vi "HFRR ADV v04 new software.vi"() -> ()   [LabVIEW 2025] (continued)
                        n2285 = property on="Coefficient of Friction" class="WFChart (strict)"("History Data"=w3332) -> ()  [unwired: 2 in, 2 out]
                        n2286 = property on="Frictional Force ( N )" class="WFChart (strict)"("History Data"=w3332) -> ()  [unwired: 2 in, 2 out]
                        n2287 = property on="Electrical Contact Resistance ( % )" class="WFChart (strict)"("History Data"=w3332) -> ()  [unwired: 2 in, 2 out]
                        n2288 = property on="Humidity ( %RH )" class="WFChart (strict)"("History Data"=w3332) -> ()  [unwired: 2 in, 2 out]
                        n2289 = property on="Stroke ( mm )" class="WFChart (strict)"("History Data"=w3333) -> ()  [unwired: 2 in, 2 out]
                        n2290 = property on="Temperature ( Deg C )" class="WFChart (strict)"("History Data"=w3332) -> ()  [unwired: 2 in, 2 out]
                        n2291 = property on="Service Password Log" class="Str"("Visible"=w3334) -> ()  [unwired: 2 in, 2 out]
                        n2292 = property on="Password 3" class="Clust (strict)"("Visible"=w3334) -> ()  [unwired: 2 in, 2 out]
                      }
                    }
                    "TEST FILE NAM,E SAVED" <- TRUE ("TEST FILE NAM,E SAVED")
                  }
                }
              }
            }
          }
        }
        n2293 = case shown="True" w2651 {
          frame False {
            n2294 = local write "tfalg"(0.0 ("tfalg")) -> ()
          }
          frame True {
            n2295 = local read "tfalg"() -> (w2796:dbl)
            n2296 = Equal?(x=w2796, y=0.0) -> (x = y?=w2797:bool)
            n2297 = case shown="True" w2797 {
              frame False {
              }
              frame True {
                n2298 = local read "Total No. of Tests"() -> (w2800:dbl)
                n2299 = local write "tfalg"(1.0 ("tfalg")) -> ()
                n2300 = local write "acq 2"(FALSE ("acq 2")) -> ()
                n2301 = Wait (ms)(milliseconds to wait=u32 200) -> ()  [unwired: 1 out]
                n2302 = Increment(x=w2800) -> (x+1=w2799:dbl)
                n2303 = local write "Total No. of Tests"(w2799) -> ()
              }
            }
          }
        }
        n2304 = local write "Test \nStatus"(w2657) -> ()
        n2305 = local write "Save"(w2657) -> ()
        n2306 = local read "Main Tab"() -> (w2614:T2)
        n2307 = case shown="True" w2638 {
          tunnel: [FALSE ("RUN") TRUE ("RUN")] -> w2637
          tunnel: [_ 1] -> w2630
          frame False {
          }
          frame True {
          }
        }
        n2308 = In Range and Coerce(upper limit=w2645, x=w2618, lower limit=w2644) -> (In Range?=w2636:bool)  [unwired: 1 out]
        n2309 = In Range and Coerce(upper limit=w2642, x=w2617, lower limit=w2643) -> (In Range?=w2634:bool)  [unwired: 1 out]
        n2310 = case shown="True" w2650 {
          frame False {
            n2311 = local read "Rt 3"() -> (w2778:bool)
            n2312 = case shown="True" w2778 {
              frame False {
              }
              frame True {
                n2313 = local write "Rt 3"(FALSE ("Rt 3")) -> ()
                n2314 = local write "Json End Flg"(TRUE ("Upld AR 2")) -> ()
              }
            }
            "Rt" <- TRUE ("Rt")
            "Rt 2" <- FALSE ("Rt")
          }
          frame True {
            n2315 = local read "Rt"() -> (w2785:bool)
            n2316 = local write "Rt 2"(TRUE ("Rt 2")) -> ()
            n2317 = case shown="True" w2785 {
              frame False {
              }
              frame True {
                w2786 = TRUE ("Upld AR 2")
                n2318 = local write "Rt"(FALSE ("Rt")) -> ()
                n2319 = local write "Upld AR"(w2786) -> ()
                n2320 = local write "Json St Flg"(w2786) -> ()
              }
            }
            "Rt 3" <- TRUE ("Rt 3")
          }
        }
        n2321 = case shown="True" w2636 {
          tunnel: [FALSE ("RUN") TRUE ("RUN")] -> w2635
          tunnel: [_ 2] -> w2629
          frame False {
          }
          frame True {
          }
        }
        n2322 = case shown="True" w2634 {
          tunnel: [FALSE ("RUN") TRUE ("RUN")] -> w2633
          tunnel: [_ 3] -> w2628
          frame False {
          }
          frame True {
          }
        }
        n2323 = case shown="\"Acquire\"" w2614 {
          tunnel: w2616 -> [_ w2847]
          frame Default {
            w2846 = 0.0 ("output")
            n2324 = local write "PID-out"(w2846) -> ()
            n2325 = local write "Frequency ( Hz )"(w2846) -> ()
          }
          frame "Acquire" {
            n2326 = stacked-sequence {
              frame #0 {
                n2327 = local read "Auto Start Test"() -> (w2849:bool)
                n2328 = case shown="True" w2849 {
                  tunnel: "RUN" -> [w2870 w2873]
                  tunnel: [w2870 w2872] -> w2850
                  frame False {
                  }
                  frame True {
                    n2329 = local read "Auto Start Temp"() -> (w2871:bool)
                    n2330 = Or(x=w2873, y=w2871) -> (x .or. y?=w2872:bool)
                  }
                }
                n2331 = local read "clk"() -> (w2869:dbl)
                n2332 = local read "Save"() -> (w2865:bool)
                n2333 = Equal?(x=w2869, y=0.0) -> (x = y?=w2866:bool)
                n2334 = And(x=w2866, y=w2865) -> (x .and. y?=w2867:bool)
                n2335 = Not(x="Engage") -> (.not. x?=w2856:bool)
                n2336 = case shown="True" w2850 {
                  tunnel: [0.0 w2890] -> w2852
                  frame False {
                    (unwired) TRUE ("Visible")
                    n2337 = local read "Auto Start Test"() -> (w2877:bool)
                    n2338 = local write "Start Time"(TRUE ("Start Time")) -> ()
                    n2339 = property on="Stroke 2" class="DigNum (strict)"("Visible"=FALSE) -> ()  [unwired: 2 in, 2 out]
                    n2340 = case shown="False" w2877 {
                      frame False {
                        n2341 = property on="Heater Button" class="Bool (strict)"("DisabledEnum"=T13."Enabled" ("Disabled")) -> ()  [unwired: 2 in, 2 out]
                        n2342 = property on="Humidity" class="Bool (strict)"("DisabledEnum"=T13."Enabled" ("Disabled")) -> ()  [unwired: 2 in, 2 out]
                      }
                      frame True {
                      }
                    }
                    n2343 = case shown="False" "TestCompFlg" {
                      frame False {
                        n2344 = local read "StartFlg"() -> (w2885:bool)
                        n2345 = case shown="True" w2885 {
                          frame False {
                          }
                          frame True {
                            n2346 = flat-sequence {
                              frame #0 {
                                n2347 = local read "EVENT LOG"() -> (w2887:string)
                                n2348 = call "Event Log.vi"("Content"="Test was interrupted", "EVENT LOG"=w2887) -> ("EVENT LOG"=w2888:string)  [unwired: 8 in, 1 out]
                                n2349 = local write "EVENT LOG"(w2888) -> ()
                              }
                              frame #1 {
                                w2889 = FALSE ("StartFlg")
                                n2350 = local write "Heater Button"(w2889) -> ()
                                n2351 = local write "StartFlg"(w2889) -> ()
                                n2352 = local write "Humidity"(w2889) -> ()
                              }
                            }
                          }
                        }
                      }
                      frame True {
                      }
                    }
                    n2353 = local write "String 14"("Test will autostart once parameters reach the set value." ("String 14")) -> ()
                  }
                  frame True {
                    (unwired) FALSE ("Visible")
                    n2354 = property on="Stroke 2" class="DigNum (strict)"("Visible"=TRUE) -> ()  [unwired: 2 in, 2 out]
                    n2355 = property on="STOP 2" class="Bool (strict)"("Disabled"=u8 2) -> ()  [unwired: 2 in, 2 out]
                    n2356 = local write "String 14"(" Running....." ("String 14")) -> ()
                    n2357 = property on="Heater Button" class="Bool (strict)"("DisabledEnum"=T13."Disabled and Grayed Out" ("Disabled")) -> ()  [unwired: 2 in, 2 out]
                    n2358 = property on="Humidity" class="Bool (strict)"("DisabledEnum"=T13."Disabled and Grayed Out" ("Disabled")) -> ()  [unwired: 2 in, 2 out]
                    n2359 = case shown="True" "Start Time" {
                      selector: "Start Time" -> [_ w2903]
                      frame False {
                      }
                      frame True {
                        n2360 = Not(x=w2903) -> (.not. x?=w2902:bool)
                        n2361 = local write "Start Time"(w2902) -> ()
                        n2362 = local read "EVENT LOG"() -> (w2904:string)
                        n2363 = call "Event Log.vi"("Content"="Test in progress", "EVENT LOG"=w2904) -> ("EVENT LOG"=w2906:string)  [unwired: 8 in, 1 out]
                        n2364 = local write "EVENT LOG"(w2906) -> ()
                      }
                    }
                    n2365 = local read "Set Hz"() -> (w2900:dbl)
                    n2366 = call <vilib>:"Uniform White Noise Waveform.vi"() -> ("signal out"=w2899:waveform(dbl))  [unwired: 10 in, 1 out]
                    n2367 = Add(x=w2900, y=w2899) -> (x+y=w2898:waveform(dbl))
                    n2368 = Multiply(x=w2898, y=ext 0.1) -> (x*y=w2890:waveform(ext))
                    "StartFlg" <- TRUE ("StartFlg")
                  }
                }
                n2369 = case shown="True" w2867 {
                  frame False {
                  }
                  frame True {
                    n2370 = local write "clk"(10.0 ("clk")) -> ()
                    n2371 = Get Date/Time In Seconds() -> (seconds since 1Jan1904=w2909:timestamp)
                    n2372 = To Double Precision Float(number=w2909) -> (double precision float=w2907:dbl)
                    n2373 = local write "acq timer"(w2907) -> ()
                    n2374 = local write "act save time"(w2907) -> ()
                  }
                }
                n2375 = call "Elapsed Time"("Time Target (s)"="Countdown", "Reset"=w2856) -> ("Elapsed Time (s)"=w2861:dbl, "Time has Elapsed"=w2859:bool)  [unwired: 10 in, 6 out]
                "Countdown 2" <- w2861
                n2376 = Subtract(x=w2861, y=2.0) -> (x-y=w2864:dbl)
                n2377 = Less?(x=w2864, y="Countdown") -> (x < y?=w2862:bool)
                n2378 = And(x=w2862, y=w2859) -> (x .and. y?=w2858:bool)
                n2379 = case shown="True" w2858 {
                  frame False {
                  }
                  frame True {
                    (unwired) dbl[] [] ("History Data")
                    n2380 = local write "Engage"(FALSE ("Engage")) -> ()
                    n2381 = local write "RUN"(TRUE ("RUN")) -> ()
                    n2382 = local read "Humidity ( %RH )"() -> (→"Rh Before":dbl)
                  }
                }
                n2383 = local read "Test \nStatus"() -> (w2854:bool)
                n2384 = Select(t=w2852, s=w2854, f=0.0) -> (s? t:f=w2853:dbl)
                n2385 = local write "Frequency ( Hz )"(w2853) -> ()
              }
              frame #1 {
                w2932 = 1000000.0 ("x")
                # "HC;1/0\nST;VALUE"
                # "Elapsed time\ncof\nstroke\nAir temp\nTemp\nHumidity"
                # "acq timer\n\nact save time"
                # "convert to microseconds"
                n2386 = local read "COUNT"() -> (w2915:i32)
                n2387 = local read "Rate"() -> (w2928:dbl)
                n2388 = Divide(x=w2932, y=w2928) -> (x/y=w2933:dbl)
                n2389 = Greater Or Equal?(x=w2915, y=250) -> (x >= y?=w2914:bool)
                n2390 = Get Date/Time In Seconds() -> (seconds since 1Jan1904=w2935:timestamp)
                n2391 = case shown="True" w2914 {
                  frame False {
                    n2392 = local read "COUNT"() -> (w2936:i32)
                    n2393 = Increment(x=w2936) -> (x+1=w2937:i32)
                    n2394 = local write "COUNT"(w2937) -> ()
                  }
                  frame True {
                    n2395 = local write "COUNT"(0 ("COUNT")) -> ()
                  }
                }
                n2396 = local read "Samplingtime 2"() -> (w2913:dbl)
                n2397 = local read "act save time"() -> (w2930:dbl)
                n2398 = Divide(x=w2933, y=w2932) -> (x/y=w2931:dbl)
                n2399 = To Double Precision Float(number=w2935) -> (double precision float=w2924:dbl)
                n2400 = Add(x=w2930, y=w2913) -> (x+y=w2929:dbl)
                n2401 = local read "acq timer"() -> (w2934:dbl)
                n2402 = local read "COUNT"() -> (w2917:i32)
                n2403 = Greater Or Equal?(x=w2924, y=w2929) -> (x >= y?=w2912:bool)
                n2404 = Multiply(x=w2931, y=w2917) -> (x*y=w2923:dbl)
                n2405 = Subtract(x=w2924, y=w2934) -> (x-y=w2926:dbl)
                n2406 = local read "Save"() -> (w2927:bool)
                n2407 = Add(x=w2926, y=w2923) -> (x+y=w2910:dbl)
                "Elapsed time 3" <- w2910
                n2408 = And(x=w2912, y=w2927) -> (x .and. y?=w2925:bool)
                n2409 = Divide(x=w2910, y=60.0) -> (x/y=w2921:dbl)
                n2410 = local read "Test \nStatus"() -> (w2911:bool)
                n2411 = local read "clk"() -> (w2918:dbl)
                n2412 = Equal?(x=w2918, y=10.0) -> (x = y?=w2920:bool)
                n2413 = case shown="True" w2925 {
                  tunnel: w2924 -> [_ w3040]
                  tunnel: [FALSE ("Boolean 2") TRUE ("Boolean 2")] -> _
                  frame False {
                  }
                  frame True {
                    w2994 = ";" ("Substring")
                    # "Pid out/\nFreq response value"
                    n2414 = local write "act save time"(w3040) -> ()
                    n2415 = local read "FILE"() -> (w2988:string)
                    n2416 = call "file check.vi"("file name in"=w2988) -> ("error out"=w2991:errorcluster, "file name out"=w2986:string)  [unwired: 9 in]
                    n2417 = call "FILE PATH CREATION.vi"("error in"=w2991, "FILE NAME :"=w2986) -> ("FILE OUT"=w2989:path)  [unwired: 8 in, 1 out]
                    n2418 = Concatenate Strings(w2986, ".dgf" ("Substring")) -> (w2990:string)
                    n2419 = local read "FF 2"() -> (→"Frictional Force ( N )" →"Frictional Force ( N )":dbl)
                    n2420 = Build Path(base path=w2989, name or relative path=w2990) -> (appended path=w2985:path)
                    n2421 = local read "COF 2"() -> (w2999:dbl)
                    "cof" <- w2999
                    "Coefficient of Friction" <- w2999
                    "COF 4" <- w2999
                    "Coefficient of Friction" <- w2999
                    n2422 = local read "TEMP"() -> (w3002:dbl)
                    "Temp" <- w3002
                    "Temperature ( Deg C )" <- w3002
                    n2423 = local read "Humidity ( %RH )"() -> (w3001:dbl)
                    "Humidity ( %RH )" <- w3001
                    "Humidity ( %RH )" <- w3001
                    n2424 = local read "Frequency ( Hz )"() -> (w3008:dbl)
                    n2425 = local read "Elapsed time"() -> (w3033:dbl)
                    n2426 = local read "AIR TEMP"() -> (w3006:dbl)
                    n2427 = local read "PID-out"() -> (w3011:dbl)
                    n2428 = local write "Temperature ( Deg C )"(w3002) -> ()
                    n2429 = Number To Fractional String(number="measured_stroke", width (-)=i16 9 ("precision (6)"), precision (6)=i16 6) -> (F-format string=w3026:string)  [unwired: 1 in]
                    n2430 = Number To Fractional String(number=w3006, width (-)=i16 9 ("precision (6)"), precision (6)=i16 3) -> (F-format string=w3025:string)  [unwired: 1 in]
                    n2431 = Number To Fractional String(number=w3002, width (-)=i16 9 ("precision (6)"), precision (6)=i16 3) -> (F-format string=w3022:string)  [unwired: 1 in]
                    n2432 = Number To Fractional String(number=w3001, width (-)=i16 9 ("precision (6)"), precision (6)=i16 3) -> (F-format string=w3019:string)  [unwired: 1 in]
                    n2433 = Number To Fractional String(number=0.0, width (-)=i16 9 ("precision (6)"), precision (6)=i16 3) -> (F-format string=w3016:string)  [unwired: 1 in]
                    n2434 = Number To Fractional String(number=w3011, width (-)=i16 9 ("precision (6)"), precision (6)=i16 3) -> (F-format string=w3012:string)  [unwired: 1 in]
                    n2435 = Number To Fractional String(number=w3008, width (-)=i16 9 ("precision (6)"), precision (6)=i16 3) -> (F-format string=w3007:string)  [unwired: 1 in]
                    n2436 = Number To Fractional String(number=w2999, width (-)=i16 9 ("precision (6)"), precision (6)=i16 6) -> (F-format string=w3034:string)  [unwired: 1 in]
                    n2437 = Number To Fractional String(number=w3033, width (-)=i16 14 ("precision (6)"), precision (6)=i16 3) -> (F-format string=w3035:string)  [unwired: 1 in]
                    n2438 = Bundle("y"=1.02, "measured_stroke"="measured_stroke", "y"=0.98) -> (w3000:cluster{"y":dbl, "measured_stroke":dbl, "y":dbl})  [unwired: 1 in]
                    n2439 = Number To Fractional String(number="Ambient Humidity :", width (-)=i16 9 ("precision (6)"), precision (6)=i16 6) -> (F-format string=w2992:string)  [unwired: 1 in]
                    n2440 = local read "RUN"() -> (w2998:bool)
                    n2441 = case shown="True" w2998 {
                      tunnel: w3000 -> [_ w3045]
                      tunnel: "measured_stroke" -> [_ w3044]
                      tunnel: "measured_stroke" -> [_ w3043]
                      tunnel: "measured_stroke" -> [_ w3042]
                      frame False {
                      }
                      frame True {
                        "Stroke ( mm )" <- w3045
                        "Stroke ( mm )" <- w3045
                        "Stroke 4" <- w3044
                        "Stroke 3" <- w3043
                        "Stroke 2" <- w3042
                      }
                    }
                    n2442 = Concatenate Strings(w3035, w2994, w3034, w2994, w3026, w2994, w3025, w2994, w3022, w2994, w3019, w2994, w3016, w2994, w3012, w2994, w3007, w2994, w2992, "\r") -> (w3032:string)
                    n2443 = call <vilib>:"Write Characters To File.vi"("append to file? (new file:F)"=TRUE, "character string"=w3032, "file path (dialog if empty)"=w2985) -> ()  [unwired: 2 in, 1 out]
                    "refresh flag" <- TRUE ("refresh flag")
                  }
                }
                n2444 = case shown="True" w2911 {
                  tunnel: w2921 -> [_ w2947]
                  tunnel: w2926 -> [_ w2957]
                  tunnel: [0.0 w2953] -> _
                  tunnel: w2920 -> [_ w2952]
                  tunnel: [0.0 w2951] -> _
                  tunnel: w2910 -> [_ w2951]
                  tunnel: w2924 -> [w2940 _]
                  frame False {
                    n2445 = local write "acq timer"(w2940) -> ()
                    n2446 = local write "Test Duration Status"(0.0 ("Test Duration Status")) -> ()
                  }
                  frame True {
                    n2447 = local read "Set Hz"() -> (w2954:dbl)
                    n2448 = local write "Elapsed time"(w2947) -> ()
                    n2449 = local read "test time"() -> (w2946:dbl)
                    n2450 = Multiply(x=w2957, y=w2954) -> (x*y=w2956:dbl)
                    n2451 = case shown="False" w2952 {
                      tunnel: w2956 -> [w2958 _]
                      tunnel: [w2958 1.0] -> w2953
                      frame False {
                        n2452 = local write "Cycles elapsed"(w2958) -> ()
                      }
                      frame True {
                      }
                    }
                    n2453 = Greater?(x=w2947, y=w2946) -> (0:w2955:bool)
                    n2454 = Subtract(x=w2946, y=w2947) -> (x-y=w2945:dbl)
                    "time" <- w2945
                    n2455 = Multiply(x=w2945, y=60.0) -> (x*y=w2944:dbl)
                    n2456 = local write "Time Remaining"(w2944) -> ()
                    n2457 = local write "Remaining Time"(w2944) -> ()
                    n2458 = case shown="True" w2955 {
                      frame False {
                      }
                      frame True {
                        n2459 = stacked-sequence {
                          frame #0 {
                            w2961 = T13."Enabled" ("Disabled")
                            w2960 = FALSE ("TEST FILE NAM,E SAVED")
                            w2964 = "" ("FILE")
                            w2965 = TRUE ("Visible")
                            n2460 = local write "Humidity"(FALSE ("Humidity")) -> ()
                            n2461 = local write "RUN"(FALSE ("OK Button 2")) -> ()
                            n2462 = local write "Heater Button"(FALSE ("Heater Button")) -> ()
                            n2463 = local write "Auto Start Test"(FALSE ("Auto Start Test")) -> ()
                            n2464 = local write "TestCompFlg"(TRUE ("StpFlg")) -> ()
                            n2465 = local read "Humidity ( %RH )"() -> (→"Rh After":dbl)
                            n2466 = property on="STOP 2" class="Bool (strict)"("Disabled"=u8 0) -> ()  [unwired: 2 in, 2 out]
                            n2467 = local read "EVENT LOG"() -> (w2970:string)
                            n2468 = call "Event Log.vi"("Content"="Test Completed", "EVENT LOG"=w2970) -> ("EVENT LOG"=w2969:string)  [unwired: 8 in, 1 out]
                            n2469 = property on="RUN" class="Bool (strict)"("Visible"=w2965) -> ()  [unwired: 2 in, 2 out]
                            n2470 = property on="Auto Start Test" class="Bool (strict)"("Visible"=w2965) -> ()  [unwired: 2 in, 2 out]
                            n2471 = local write "Batch Ref Num :"(w2964) -> ()
                            n2472 = local write "FILE"(w2964) -> ()
                            n2473 = local write "EVENT LOG"(w2969) -> ()
                            n2474 = local write "TEST FILE NAM,E SAVED"(w2960) -> ()
                            n2475 = local write "Fuel Discription :"(w2964) -> ()
                            n2476 = local write "START TEMP"(w2960) -> ()
                            n2477 = local write "Remarks :"(w2964) -> ()
                            n2478 = local write "Main Dashboard Buttons"(T1."Imaging" ("Main Dashboard Buttons")) -> ()
                            n2479 = local write "Main Tab"(T2."Adv Scar" ("Main Tab")) -> ()
                            n2480 = property on="FRICVALZ 2" class="Bool (strict)"("DisabledEnum"=w2961) -> ()  [unwired: 2 in, 2 out]
                            n2481 = property on="FRICVALZ 3" class="Bool (strict)"("DisabledEnum"=w2961) -> ()  [unwired: 2 in, 2 out]
                            n2482 = property on="FRICVALZ 4" class="Bool (strict)"("DisabledEnum"=w2961) -> ()  [unwired: 2 in, 2 out]
                          }
                          frame #1 {
                            n2483 = Wait (ms)(milliseconds to wait=u32 1500) -> ()  [unwired: 1 out]
                          }
                          frame #2 {
                            n2484 = local write "Command"("VC;0") -> ()
                          }
                          frame #3 {
                            n2485 = Wait (ms)(milliseconds to wait=u32 1500) -> ()  [unwired: 1 out]
                          }
                          frame #4 {
                            n2486 = local write "Command"("ST;0") -> ()
                          }
                          frame #5 {
                            n2487 = Wait (ms)(milliseconds to wait=u32 1500) -> ()  [unwired: 1 out]
                          }
                          frame #6 {
                            n2488 = local write "Command"("HE;0") -> ()
                          }
                        }
                      }
                    }
                    n2489 = Divide(x=w2947, y=w2946) -> (x/y=w2950:dbl)
                    n2490 = Multiply(x=w2950, y=100.0) -> (x*y=w2948:dbl)
                    n2491 = local write "Test Duration Status"(w2948) -> ()
                  }
                }
              }
              frame #2 {
                n2492 = case shown="True" "Heater Button" {
                  tunnel: [0.0 ("output") w3068] -> w3046
                  frame False {
                    w3049 = TRUE ("tmpchk")
                    n2493 = local read "TEMP"() -> (w3050:dbl)
                    n2494 = local write "Temp ini"(w3050) -> ()
                    n2495 = local write "Reset 4"(w3049) -> ()
                    n2496 = local write "tmpchk"(w3049) -> ()
                    n2497 = local write "reinit"(TRUE ("reinit")) -> ()
                    n2498 = local write "manual temp log"(TRUE ("manual temp log")) -> ()
                  }
                  frame True {
                    # "Logic to turn off\nthe heater when \ntemp is not rising.\nTime - 60 sec\nDelta t- 5°c"
                    n2499 = local read "Temp ini"() -> (w3057:dbl)
                    n2500 = local read "Auto Start Test"() -> (w3053:bool)
                    n2501 = Less?(x=w3057, y=53.0) -> (x < y?=w3055:bool)
                    n2502 = case shown="False" w3053 {
                      frame False {
                        n2503 = local read "Set Temp"() -> (w3077:dbl)
                        n2504 = local read "TEMP"() -> (w3076:dbl)
                        n2505 = Subtract(x=w3077, y=w3076) -> (x-y=w3075:dbl)
                        n2506 = Absolute Value(x=w3075) -> (abs(x)=w3074:dbl)
                        n2507 = Less?(x=w3074, y=0.5) -> (x < y?=w3072:bool)
                        n2508 = case shown="True" w3072 {
                          tunnel: "manual temp log" -> [_ w3078]
                          frame False {
                          }
                          frame True {
                            n2509 = case shown="True" w3078 {
                              selector: w3078 -> [_ w3079]
                              frame False {
                              }
                              frame True {
                                # "#Event log"
                                n2510 = Not(x=w3079) -> (.not. x?=w3080:bool)
                                n2511 = local write "manual temp log"(w3080) -> ()
                                n2512 = local read "EVENT LOG"() -> (w3083:string)
                                n2513 = call "Event Log.vi"("Content"="Target Temperature reached", "EVENT LOG"=w3083) -> ("EVENT LOG"=w3082:string)  [unwired: 8 in, 1 out]
                                n2514 = local write "EVENT LOG"(w3082) -> ()
                              }
                            }
                          }
                        }
                      }
                      frame True {
                        n2515 = local write "manual temp log"(TRUE ("manual temp log")) -> ()
                      }
                    }
                    n2516 = And(x="tmpchk", y=w3055) -> (x .and. y?=w3058:bool)
                    n2517 = case shown="True" w3058 {
                      frame False {
                      }
                      frame True {
                        n2518 = call "Elapsed Time8"("Time Target (s)"=300.0, "Reset"="Reset 4") -> ("Time has Elapsed"=w3085:bool)  [unwired: 10 in, 7 out]
                        n2519 = flat-sequence {
                          tunnel: w3085 -> [_]
                          frame #0 {
                            n2520 = local write "Reset 4"(FALSE ("Reset 4")) -> ()
                          }
                        }
                        n2521 = case shown="True" w3085 {
                          frame False {
                          }
                          frame True {
                            n2522 = local read "Temp ini"() -> (w3092:dbl)
                            n2523 = Add(x=w3092, y=5.0) -> (x+y=w3090:dbl)
                            n2524 = local read "TEMP"() -> (w3093:dbl)
                            n2525 = Greater?(x=w3093, y=w3090) -> (0:w3091:bool)
                            n2526 = case shown="False" w3091 {
                              frame False {
                                n2527 = local write "Heater Button"(FALSE ("Heater Button")) -> ()
                              }
                              frame True {
                                n2528 = local write "tmpchk"(FALSE ("tmpchk")) -> ()
                              }
                            }
                          }
                        }
                      }
                    }
                    n2529 = local read "Set Temp"() -> (w3066:dbl)
                    n2530 = local read "TEMP"() -> (w3060:dbl)
                    n2531 = call-poly <vilib>:"PID.vi"("reinitialize? (F)"="reinit", "dt (s)"=-1.0, "process variable"=w3060, "setpoint"=w3066) -> ("output"=w3063:dbl)  [unwired: 6 in, 1 out]
                    n2532 = Subtract(x=w3066, y=w3060) -> (x-y=w3067:dbl)
                    n2533 = Add(x=w3066, y=0.5) -> (x+y=w3064:dbl)
                    n2534 = Greater Or Equal?(x=w3060, y=w3064) -> ()  [unwired: 1 out]
                    n2535 = Select(t=0.0, s=FALSE, f=w3063) -> (s? t:f=w3062:dbl)
                    "PID output" <- w3062
                    n2536 = flat-sequence {
                      tunnel: w3062 -> [w3096]
                      tunnel: [w3096] -> w3068
                      frame #0 {
                        n2537 = local write "reinit"(FALSE ("reinit")) -> ()
                      }
                    }
                    n2538 = Bundle(w3067, "output"=w3062, "TEMP"=w3060) -> ()  [unwired: 1 in, 1 out]
                  }
                }
                "PID-out" <- w3046
              }
              frame #3 {
                n2539 = local read "TEMP"() -> (w3098:dbl)
                n2540 = Greater Or Equal?(x=w3098, y="Set Temp 2") -> (x >= y?=w3103:bool)
                n2541 = case shown="True" w3103 {
                  tunnel: [FALSE TRUE] -> w3101
                  frame False {
                  }
                  frame True {
                  }
                }
                "Status 13" <- w3101
                n2542 = And(x=w3101, y="trip1 8") -> (x .and. y?=w3100:bool)
                n2543 = case shown="True" w3100 {
                  frame False {
                    n2544 = local write "Heater Trip Temp"(TRUE ("Heater Trip Temp")) -> ()
                  }
                  frame True {
                    w3106 = FALSE ("OK Button 2")
                    n2545 = case shown="True" "Heater Trip Temp" {
                      selector: "Heater Trip Temp" -> [_ w3108]
                      frame False {
                      }
                      frame True {
                        n2546 = Not(x=w3108) -> (.not. x?=w3107:bool)
                        n2547 = local read "EVENT LOG"() -> (w3111:string)
                        n2548 = local write "Heater Trip Temp"(w3107) -> ()
                        n2549 = call "Event Log.vi"("Content"="Heater Trip", "EVENT LOG"=w3111) -> ("EVENT LOG"=w3110:string)  [unwired: 8 in, 1 out]
                        n2550 = local write "EVENT LOG"(w3110) -> ()
                      }
                    }
                    n2551 = local write "RUN"(w3106) -> ()
                    n2552 = property on="Auto Start Test" class="Bool (strict)"("Value"=w3106) -> ()  [unwired: 2 in, 2 out]
                    n2553 = local write "Heater Button"(w3106) -> ()
                  }
                }
              }
            }
            n2554 = case shown="False" w2847 {
              frame False {
                n2555 = disable-structure shown="Disabled" {
                  frame Disabled {
                    n2556 = stacked-sequence {
                      frame #0 {
                        n2557 = local write "RUN"(FALSE ("OK Button 2")) -> ()
                      }
                      frame #1 {
                      }
                    }
                  }
                  frame Enabled {
                  }
                }
              }
              frame True {
              }
            }
          }
        }
        n2558 = local read "airtempflg"() -> (w2639:bool)
        n2559 = Or(x=w2639, y=w2637) -> (x .or. y?=w2640:bool)
        n2560 = Insert Into Array(array=string[] ["Air Temperature has reached set value,", "Humidity has reached set value,", "Sample Temperaturehas reached set value,", ""], index=0, new element="") -> (w2625:string[])
        n2561 = Build Array(w2630, w2629, w2628) -> (w2626:i32[])
        n2562 = disable-structure shown="Disabled" {
          disable-tunnel: w2640 -> [w2717 _]
          disable-tunnel: w2635 -> [w2716 _]
          disable-tunnel: w2633 -> [w2715 _]
          frame Disabled {
            n2563 = Compound Arithmetic op=AND(w2717, w2716, w2715) -> ()  [unwired: 1 out]
            n2564 = case shown="True" {
              selector: _ -> [_ _]
              frame False {
              }
              frame True {
                w2718 = FALSE ("autostrtflg")
                n2565 = local write "RUN"(TRUE ("RUN")) -> ()
                n2566 = local write "autostrtflg"(w2718) -> ()
                n2567 = local write "autostart"(w2718) -> ()
                n2568 = local write "String 14"(" Running....." ("String 14")) -> ()
              }
            }
          }
          frame Enabled {
          }
        }
        n2569 = for {
          tunnel: w2626 -> [w2768] mode=indexing
          tunnel: w2625 -> [w2767]
          shift-right: [w2764] -> w2624
          shift-left: "" -> [w2766]
          n2570 = Index Array(array=w2767, index=w2768) -> (element=w2765:string)
          n2571 = Concatenate Strings(w2765, w2766) -> (w2764:string)
        }
        n2572 = local write "autostart 2"(w2624) -> ()
        n2573 = local read "Reset Graph"() -> (w2613:bool)
        n2574 = case shown="True" w2613 {
          selector: w2613 -> [_ w2667]
          frame False {
          }
          frame True {
            w2681 = 0.0 ("X Scale.Range:Maximum")
            n2575 = Not(x=w2667) -> (.not. x?=w2666:bool)
            n2576 = local write "Reset Graph"(w2666) -> ()
            n2577 = property on="Electrical Contact Resistance ( % )" class="WFChart (strict)"("XScale.Maximum"=600.0 ("X Scale.Range:Maximum"), "XScale.Minimum"=0.0 ("X Scale.Range:Minimum"), "YScale.Maximum"=100.0 ("Y Scale.Range:Maximum"), "YScale.Minimum"=0.0 ("Y Scale.Range:Minimum")) -> ()  [unwired: 2 in, 2 out]
            n2578 = property on="Frictional Force ( N )" class="WFChart (strict)"("XScale.Maximum"=600.0 ("X Scale.Range:Maximum"), "XScale.Minimum"=0.0 ("X Scale.Range:Minimum"), "YScale.Maximum"=100.0 ("Y Scale.Range:Maximum"), "YScale.Minimum"=0.0 ("Y Scale.Range:Minimum")) -> ()  [unwired: 2 in, 2 out]
            n2579 = property on="Temperature ( Deg C )" class="WFChart (strict)"("XScale.Maximum"=600.0 ("X Scale.Range:Maximum"), "XScale.Minimum"=0.0 ("X Scale.Range:Minimum"), "YScale.Maximum"=100.0 ("Y Scale.Range:Maximum"), "YScale.Minimum"=0.0 ("Y Scale.Range:Minimum")) -> ()  [unwired: 2 in, 2 out]
            n2580 = property on="Humidity ( %RH )" class="WFChart (strict)"("XScale.Maximum"=600.0 ("X Scale.Range:Maximum"), "XScale.Minimum"=0.0 ("X Scale.Range:Minimum"), "YScale.Maximum"=100.0 ("Y Scale.Range:Maximum"), "YScale.Minimum"=0.0 ("Y Scale.Range:Minimum")) -> ()  [unwired: 2 in, 2 out]
            n2581 = property on="Stroke ( mm )" class="WFChart (strict)"("XScale.Maximum"=600.0 ("X Scale.Range:Maximum"), "XScale.Minimum"=0.0 ("X Scale.Range:Minimum"), "YScale.Maximum"=100.0 ("Y Scale.Range:Maximum"), "YScale.Minimum"=0.0 ("Y Scale.Range:Minimum")) -> ()  [unwired: 2 in, 2 out]
            n2582 = property on="Coefficient of Friction" class="WFChart (strict)"("XScale.Maximum"=600.0 ("X Scale.Range:Maximum"), "XScale.Minimum"=0.0 ("X Scale.Range:Minimum"), "YScale.Maximum"=100.0 ("Y Scale.Range:Maximum"), "YScale.Minimum"=0.0 ("Y Scale.Range:Minimum")) -> ()  [unwired: 2 in, 2 out]
            n2583 = property on="Electrical Contact Resistance ( % )" class="WFChart (strict)"("XScale.Minimum"=0.0 ("X Scale.Range:Minimum"), "XScale.Maximum"=600.0 ("X Scale.Range:Maximum"), "YScale.Minimum"=0.0 ("Y Scale.Range:Minimum"), "YScale.Maximum"=100.0 ("Y Scale.Range:Maximum")) -> ()  [unwired: 2 in, 2 out]
            n2584 = property on="Temperature ( Deg C )" class="WFChart (strict)"("XScale.Minimum"=0.0 ("X Scale.Range:Minimum"), "XScale.Maximum"=600.0 ("X Scale.Range:Maximum"), "YScale.Minimum"=0.0 ("Y Scale.Range:Minimum"), "YScale.Maximum"=100.0 ("Y Scale.Range:Maximum")) -> ()  [unwired: 2 in, 2 out]
            n2585 = property on="Coefficient of Friction" class="WFChart (strict)"("XScale.Minimum"=0.0 ("X Scale.Range:Minimum"), "XScale.Maximum"=600.0 ("X Scale.Range:Maximum"), "YScale.Maximum"=1.0 ("X Scale.Range:Minimum"), "YScale.Minimum"=0.0 ("X Scale.Range:Minimum")) -> ()  [unwired: 2 in, 2 out]
            n2586 = property on="Frictional Force ( N )" class="WFChart (strict)"("XScale.Maximum"=600.0 ("X Scale.Range:Maximum"), "XScale.Minimum"=w2681, "YScale.Maximum"=10.0 ("Y Scale.Range:Maximum"), "YScale.Minimum"=w2681) -> ()  [unwired: 2 in, 2 out]
            n2587 = property on="Stroke ( mm )" class="WFChart (strict)"("XScale.Maximum"=600.0 ("X Scale.Range:Maximum"), "XScale.Minimum"=0.0 ("X Scale.Range:Minimum"), "YScale.Maximum"=100.0 ("Y Scale.Range:Maximum"), "YScale.Minimum"=0.0 ("Y Scale.Range:Minimum")) -> ()  [unwired: 2 in, 2 out]
            n2588 = property on="Humidity ( %RH )" class="WFChart (strict)"("XScale.Maximum"=600.0 ("X Scale.Range:Maximum"), "XScale.Minimum"=0.0 ("X Scale.Range:Minimum"), "YScale.Maximum"=100.0 ("Y Scale.Range:Maximum"), "YScale.Minimum"=0.0 ("Y Scale.Range:Minimum")) -> ()  [unwired: 2 in, 2 out]
          }
        }
      }
      frame "Compare Files" {
        # "Elapsed time\ncof\nstroke\nAir temp\nTemp\nHumidity"
        n2589 = case shown="True" "RSTV1 2" {
          frame False {
          }
          frame True {
            n2590 = property on="Humidity ( %RH )" class="XYGraph (strict)"("Y Scale.Display Format:Precision"=u8 0 ("Y Scale.Format & Precision:Precision")) -> ()  [unwired: 2 in, 2 out]
            n2591 = property on="Humidity ( %RH )" class="XYGraph (strict)"("X Scale.Range:Minimum"=0.0, "X Scale.Range:Maximum"=75.0, "Y Scale.Range:Minimum"=48.0, "Y Scale.Range:Maximum"=58.0) -> ()  [unwired: 2 in, 2 out]
          }
        }
        n2592 = case shown="True" "RST CP 2" {
          frame False {
          }
          frame True {
            n2593 = property on="XY Graph 13" class="XYGraph (strict)"("Y Scale.Display Format:Precision"=u8 0 ("Y Scale.Format & Precision:Precision")) -> ()  [unwired: 2 in, 2 out]
            n2594 = property on="XY Graph 13" class="XYGraph (strict)"("X Scale.Range:Minimum"=0.0, "X Scale.Range:Maximum"=75.0, "Y Scale.Range:Minimum"=0.0, "Y Scale.Range:Maximum"=100.0) -> ()  [unwired: 2 in, 2 out]
          }
        }
        n2595 = case shown="True" "RST CP" {
          frame False {
          }
          frame True {
            n2596 = property on="Sample Temperature ( °C )" class="XYGraph (strict)"("Y Scale.Display Format:Precision"=u8 2 ("Y Scale.Format & Precision:Precision")) -> ()  [unwired: 2 in, 2 out]
            n2597 = property on="Sample Temperature ( °C )" class="XYGraph (strict)"("X Scale.Range:Minimum"=0.0, "X Scale.Range:Maximum"=75.0, "Y Scale.Range:Minimum"=58.0, "Y Scale.Range:Maximum"=62.0) -> ()  [unwired: 2 in, 2 out]
          }
        }
        n2598 = case shown="True" "RSTV1 3" {
          frame False {
          }
          frame True {
            n2599 = property on="Air Temperature  ( °C )" class="XYGraph (strict)"("Y Scale.Display Format:Precision"=u8 2 ("Y Scale.Format & Precision:Precision")) -> ()  [unwired: 2 in, 2 out]
            n2600 = property on="Air Temperature  ( °C )" class="XYGraph (strict)"("X Scale.Range:Minimum"=0.0 ("Y Scale.Range:Minimum"), "X Scale.Range:Maximum"=75.0 ("Y Scale.Range:Maximum"), "Y Scale.Range:Minimum"=20.0 ("X Scale.Range:Minimum"), "Y Scale.Range:Maximum"=26.0 ("X Scale.Range:Maximum")) -> ()  [unwired: 2 in, 2 out]
          }
        }
        n2601 = case shown="True" "RSTV1 4" {
          frame False {
          }
          frame True {
            n2602 = property on="Stroke ( mm )" class="XYGraph (strict)"("Y Scale.Display Format:Precision"=u8 2 ("Y Scale.Format & Precision:Precision")) -> ()  [unwired: 2 in, 2 out]
            n2603 = property on="Stroke ( mm )" class="XYGraph (strict)"("X Scale.Range:Minimum"=0.0 ("Y Scale.Range:Maximum"), "X Scale.Range:Maximum"=75.0 ("X Scale.Range:Minimum"), "Y Scale.Range:Minimum"=0.98, "Y Scale.Range:Maximum"=1.02) -> ()  [unwired: 2 in, 2 out]
          }
        }
        n2604 = case shown="True" "rstv2" {
          frame False {
          }
          frame True {
            n2605 = property on="Coefficient Of Friction" class="XYGraph (strict)"("Y Scale.Display Format:Precision"=u8 3 ("Y Scale.Format & Precision:Precision")) -> ()  [unwired: 2 in, 2 out]
            n2606 = property on="Coefficient Of Friction" class="XYGraph (strict)"("X Scale.Range:Minimum"=0.0 ("Y Scale.Range:Maximum"), "X Scale.Range:Maximum"=75.0, "Y Scale.Range:Minimum"=0.0, "Y Scale.Range:Maximum"=1.0 ("X Scale.Range:Minimum")) -> ()  [unwired: 2 in, 2 out]
          }
        }
        n2607 = case shown="True" "RST CP 3" {
          frame False {
          }
          frame True {
            n2608 = property on="Air Temp ( °C ) vs Humidity ( % RH )" class="XYGraph (strict)"("X Scale.Range:Minimum"=18.0, "X Scale.Range:Maximum"=28.0 ("X Scale.Range:Minimum"), "Y Scale.Range:Minimum"=30.0 ("X Scale.Range:Minimum"), "Y Scale.Range:Maximum"=70.0 ("X Scale.Range:Minimum")) -> ()  [unwired: 2 in, 2 out]
          }
        }
        n2609 = case shown="True" "OPEN 1" {
          frame False {
          }
          frame True {
            (unwired) 0  # existing file
            w3387 = "Choose a datalog file to open"  # prompt
            n2610 = local write "OPEN 1"(FALSE ("OPEN 1")) -> ()
            n2611 = String To Path(string="C:\\LAB-IQ\\Data\\") -> (path=w3372:path)
            n2612 = File Dialog(6:"*.dgf" ("pattern"), 7:w3387, 11:w3372) -> (0:w3370:errorcluster, 3:w3378:path)  [unwired: 4 in, 2 out]
            n2613 = Unbundle(w3370) -> ()  [unwired: 3 out]
            n2614 = Strip Path(path=w3378) -> (name=w3377:string)  [unwired: 1 out]
            n2615 = Path To String(path=w3378) -> (string=w3373:string)
            "string1" <- w3373
            n2616 = Match Pattern(string=w3377, regular expression=".dgf") -> (before substring=→"String Control":string)  [unwired: 1 in, 3 out]
            n2617 = Match Pattern(string=w3373, regular expression=".dgf" ("substring (\"\")")) -> (before substring=w3383:string)  [unwired: 1 in, 3 out]
            n2618 = Concatenate Strings(w3383, ".duf" ("Substring")) -> (w3379:string)
            n2619 = String To Path(string=w3379) -> (path=w3384:path)
            n2620 = call <vilib>:"Read Characters From File.vi"("file path (dialog if empty)"=w3384, "start of read offset (chars.:0)"=60 ("start of read offset (chars.: 0)")) -> ("character string"=→"String Control 2":string)  [unwired: 4 in, 3 out]
          }
        }
        n2621 = case shown="True" "OPEN 2" {
          frame False {
          }
          frame True {
            (unwired) 0  # existing file
            w3405 = "Choose a datalog file to open"  # prompt
            n2622 = local write "OPEN 2"(FALSE ("OPEN 1")) -> ()
            n2623 = String To Path(string="C:\\LAB-IQ\\Data\\") -> (path=w3390:path)
            n2624 = File Dialog(6:"*.dgf" ("pattern"), 7:w3405, 11:w3390) -> (0:w3388:errorcluster, 3:w3396:path)  [unwired: 4 in, 2 out]
            n2625 = Unbundle(w3388) -> ()  [unwired: 3 out]
            n2626 = Strip Path(path=w3396) -> (name=w3394:string)  [unwired: 1 out]
            n2627 = Path To String(path=w3396) -> (string=w3391:string)
            "string1 2" <- w3391
            n2628 = Match Pattern(string=w3394, regular expression=".dgf") -> (before substring=→"String Control 3":string)  [unwired: 1 in, 3 out]
            n2629 = Match Pattern(string=w3391, regular expression=".dgf" ("substring (\"\")")) -> (before substring=w3402:string)  [unwired: 1 in, 3 out]
            n2630 = Concatenate Strings(w3402, ".duf" ("Substring")) -> (w3399:string)
            n2631 = String To Path(string=w3399) -> (path=w3397:path)
            n2632 = call <vilib>:"Read Characters From File.vi"("file path (dialog if empty)"=w3397, "start of read offset (chars.:0)"=60 ("start of read offset (chars.: 0)")) -> ("character string"=→"String Control 4":string)  [unwired: 4 in, 3 out]
          }
        }
        n2633 = case shown="True" "OPEN 3" {
          frame False {
          }
          frame True {
            (unwired) 0  # existing file
            w3423 = "Choose a datalog file to open"  # prompt
            n2634 = local write "OPEN 3"(FALSE ("OPEN 1")) -> ()
            n2635 = String To Path(string="C:\\LAB-IQ\\Data\\") -> (path=w3408:path)
            n2636 = File Dialog(6:"*.dgf" ("pattern"), 7:w3423, 11:w3408) -> (0:w3406:errorcluster, 3:w3414:path)  [unwired: 4 in, 2 out]
            n2637 = Unbundle(w3406) -> ()  [unwired: 3 out]
            n2638 = Strip Path(path=w3414) -> (name=w3412:string)  [unwired: 1 out]
            n2639 = Path To String(path=w3414) -> (string=w3409:string)
            "string1 3" <- w3409
            n2640 = Match Pattern(string=w3412, regular expression=".dgf") -> (before substring=→"String Control 5":string)  [unwired: 1 in, 3 out]
            n2641 = Match Pattern(string=w3409, regular expression=".dgf" ("substring (\"\")")) -> (before substring=w3419:string)  [unwired: 1 in, 3 out]
            n2642 = Concatenate Strings(w3419, ".duf" ("Substring")) -> (w3416:string)
            n2643 = String To Path(string=w3416) -> (path=w3420:path)
            n2644 = call <vilib>:"Read Characters From File.vi"("file path (dialog if empty)"=w3420, "start of read offset (chars.:0)"=60 ("start of read offset (chars.: 0)")) -> ("character string"=→"String Control 6":string)  [unwired: 4 in, 3 out]
          }
        }
        n2645 = case shown="True" "OPEN 4" {
          frame False {
          }
          frame True {
            (unwired) 0  # existing file
            w3441 = "Choose a datalog file to open"  # prompt
            n2646 = local write "OPEN 4"(FALSE ("OPEN 1")) -> ()
            n2647 = String To Path(string="C:\\LAB-IQ\\Data\\") -> (path=w3426:path)
            n2648 = File Dialog(6:"*.dgf" ("pattern"), 7:w3441, 11:w3426) -> (0:w3424:errorcluster, 3:w3432:path)  [unwired: 4 in, 2 out]
            n2649 = Unbundle(w3424) -> ()  [unwired: 3 out]
            n2650 = Strip Path(path=w3432) -> (name=w3430:string)  [unwired: 1 out]
            n2651 = Path To String(path=w3432) -> (string=w3427:string)
            "string1 4" <- w3427
            n2652 = Match Pattern(string=w3430, regular expression=".dgf") -> (before substring=→"String Control 7":string)  [unwired: 1 in, 3 out]
            n2653 = Match Pattern(string=w3427, regular expression=".dgf" ("substring (\"\")")) -> (before substring=w3437:string)  [unwired: 1 in, 3 out]
            n2654 = Concatenate Strings(w3437, ".duf" ("Substring")) -> (w3434:string)
            n2655 = String To Path(string=w3434) -> (path=w3438:path)
            n2656 = call <vilib>:"Read Characters From File.vi"("file path (dialog if empty)"=w3438, "start of read offset (chars.:0)"=60 ("start of read offset (chars.: 0)")) -> ("character string"=→"String Control 8":string)  [unwired: 4 in, 3 out]
          }
        }
      }
      frame "About" {
        # "Elapsed time\ncof\nstroke\nmean pos\nTemp\nHumidity"
        n2657 = disable-structure shown="Disabled" {
          frame Disabled {
            n2658 = case shown="True" "Export" {
              frame False {
              }
              frame True {
                w3463 = "                                      " ("string")
                w3465 = "\r"
                (unwired) i16 6 ("width (-)")
                w3542 = "\r"
                w3474 = "\r"
                n2659 = local write "Export"(FALSE ("Export")) -> ()
                n2660 = local read "String 29"() -> (w3511:string)
                n2661 = local read "String 34"() -> (w3499:string)
                n2662 = local read "String 35"() -> (w3494:string)
                n2663 = local read "String 37"() -> (w3490:string)
                n2664 = local read "String 36"() -> (w3487:string)
                n2665 = local read "String 38"() -> (w3484:string)
                n2666 = local read "String 39"() -> (w3481:string)
                n2667 = Match Pattern(string=w3511, regular expression=".dwm") -> (before substring=w3507:string)  [unwired: 1 in, 3 out]
                "before substring" <- w3507
                n2668 = local read "S 38"() -> (w3502:string)
                n2669 = local read "S 39"() -> (w3495:string)
                n2670 = local read "Temperature before test 2"() -> (w3531:dbl)
                n2671 = local read "Temperature after test 2"() -> (w3536:dbl)
                n2672 = local read "Humidity before test 2"() -> (w3517:dbl)
                n2673 = local read "Humidity after test 2"() -> (w3532:dbl)
                n2674 = local read "MWSD 2"() -> (w3528:dbl)
                n2675 = local read "WS1.4 2"() -> (w3544:dbl)
                n2676 = local read "HCF 2"() -> (w3540:dbl)
                n2677 = local read "AVP 2"() -> (w3529:dbl)
                n2678 = Concatenate Strings("1," ("string"), w3502) -> (w3501:string)
                n2679 = Concatenate Strings("2," ("string"), w3499) -> (w3498:string)
                n2680 = Concatenate Strings("3," ("string"), w3495) -> (w3497:string)
                n2681 = Concatenate Strings("4," ("string"), w3494) -> (w3493:string)
                n2682 = Concatenate Strings("5," ("string"), w3490) -> (w3491:string)
                n2683 = Concatenate Strings("6," ("string"), w3487) -> (w3488:string)
                n2684 = Concatenate Strings("7," ("string"), w3484) -> (w3485:string)
                n2685 = Concatenate Strings("8," ("string"), w3481) -> (w3482:string)
                n2686 = local read "Sample ID"() -> (w3549:string)
                n2687 = case shown="\"xlx\"" "Select File Type" {
                  tunnel: w3507 -> [w3552 w3554 w3556]
                  tunnel: [w3550 w3555 w3557] -> w3506
                  frame "xlx" {
                    n2688 = Concatenate Strings(w3552, ".xls" ("string")) -> (w3550:string)
                  }
                  frame "csv" {
                    n2689 = Concatenate Strings(w3554, ".csv" ("string")) -> (w3555:string)
                  }
                  frame "txt" {
                    n2690 = Concatenate Strings(w3556, ".txt" ("string")) -> (w3557:string)
                  }
                }
                n2691 = local read "Test Date"() -> (w3548:string)
                n2692 = local read "String 45"() -> (w3462:string)
                n2693 = local read "String 31"() -> (w3547:string)
                n2694 = local read "String 32"() -> (w3546:string)
                n2695 = local read "TITTLE"() -> (w3470:string)
                n2696 = Number To Fractional String(number=w3517, width (-)=i16 6, precision (6)=i16 2) -> (F-format string=w3516:string)  [unwired: 1 in]
                n2697 = Number To Fractional String(number=w3531, width (-)=i16 6, precision (6)=i16 2) -> (F-format string=w3537:string)  [unwired: 1 in]
                n2698 = Number To Fractional String(number=w3532, width (-)=i16 6, precision (6)=i16 2) -> (F-format string=w3530:string)  [unwired: 1 in]
                n2699 = Number To Fractional String(number=w3536, width (-)=i16 6, precision (6)=i16 2) -> (F-format string=w3535:string)  [unwired: 1 in]
                n2700 = Number To Fractional String(number=w3528, width (-)=i16 6, precision (6)=i16 2) -> (F-format string=w3526:string)  [unwired: 1 in]
                n2701 = Number To Fractional String(number=w3529, width (-)=i16 6, precision (6)=i16 2) -> (F-format string=w3527:string)  [unwired: 1 in]
                n2702 = Number To Fractional String(number=w3540, width (-)=i16 6, precision (6)=i16 2) -> (F-format string=w3541:string)  [unwired: 1 in]
                n2703 = Number To Fractional String(number=w3544, precision (6)=i16 2) -> (F-format string=w3545:string)  [unwired: 2 in]
                n2704 = local read "s.NO"() -> (w3464:string)
                n2705 = Concatenate Strings("=" ("string"), w3470) -> (w3469:string)
                n2706 = Concatenate Strings("S.No," ("string"), "                                       Parameters" ("string")) -> (w3475:string)
                n2707 = Concatenate Strings(w3542, w3501, w3516, w3542, w3498, w3537, w3542, w3497, w3530, w3542, w3493, w3535, w3542, w3491, w3526, w3542, w3488, w3527, w3542, w3485, w3541, w3542, w3482, w3545) -> (w3504:string)
                n2708 = Concatenate Strings(w3474, "," ("string"), w3462, w3464, w3463, w3546, w3549, w3463, w3547, w3548, w3474) -> (w3472:string)
                n2709 = local read "Tested by"() -> (w3478:string)
                n2710 = local read "String 33"() -> (w3479:string)
                n2711 = Concatenate Strings("," ("string"), "                                                                             " ("string")) -> (w3467:string)
                n2712 = Concatenate Strings(w3469, w3465, w3472, w3465, w3475, w3504, w3465, w3467, w3479, w3478) -> (→"export":string)
                n2713 = String To Path(string=w3506) -> (path=w3513:path)
                n2714 = local read "export"() -> (w3508:string)
                n2715 = call <vilib>:"Write Characters To File.vi"("append to file? (new file:F)"=FALSE, "character string"=w3508, "file path (dialog if empty)"=w3513) -> ()  [unwired: 2 in, 1 out]
              }
            }
          }
          frame Enabled {
          }
        }
        n2716 = case shown="True" "OK Button 17" {
          frame False {
          }
          frame True {
            (unwired) 0  # existing file
            w3766 = "Choose a datalog file to open"  # prompt
            n2717 = local write "OK Button 17"(FALSE ("OK Button 17")) -> ()
            n2718 = local read "String"() -> (w3761:string)
            n2719 = String To Path(string=w3761) -> (path=w3762:path)
            n2720 = File Dialog(6:"*.duf" ("pattern"), 7:w3766, 11:w3762) -> (0:w3753:errorcluster, 3:w3772:path)  [unwired: 4 in, 2 out]
            n2721 = Unbundle(w3753) -> ()  [unwired: 3 out]
            n2722 = Open/Create/Replace File "Open File"(file path (use dialog)=w3772) -> (refnum out=w3764:refnum<file>)  [unwired: 5 in, 2 out]
            n2723 = Strip Path(path=w3772) -> (name=w3770:string)  [unwired: 1 out]
            n2724 = Path To String(path=w3772) -> (string=w3755:string)
            n2725 = while {
              tunnel: w3764 -> [w3776]
              i -> [w3773]
              stop <- w3774 continue-if-true
              (unwired) TRUE ("line mode (F)")
              n2726 = Read from Text File "Read File"(file (use dialog)=w3776) -> (text=w3775:string)  [unwired: 3 in, 3 out]
              n2727 = local write "Numeric 16"(w3773) -> ()
              n2728 = String Length(string=w3775) -> (length=w3778:i32)
              n2729 = Greater?(x=w3778, y=1) -> (0:w3774:bool)
            }
            n2730 = local write "String 29"(w3755) -> ()
